vi "Serialize.vi"(7 "MsgSerializer":refnum<class "MsgSerializer.JSON.lvclass">, 8 "error in (no error)":errorcluster, 11 "Value":variant) -> (0 "error out":errorcluster, 3 "Serialized Message":string)   [LabVIEW 2020, in "Caraya.lvlib" / "MsgSerializer.JSON.lvclass"]
uses:
  MsgSerializer.JSON.lvclass
  <vilib>/Utility/VariantDataType/VariantType.lvlib
  Caraya.lvlib
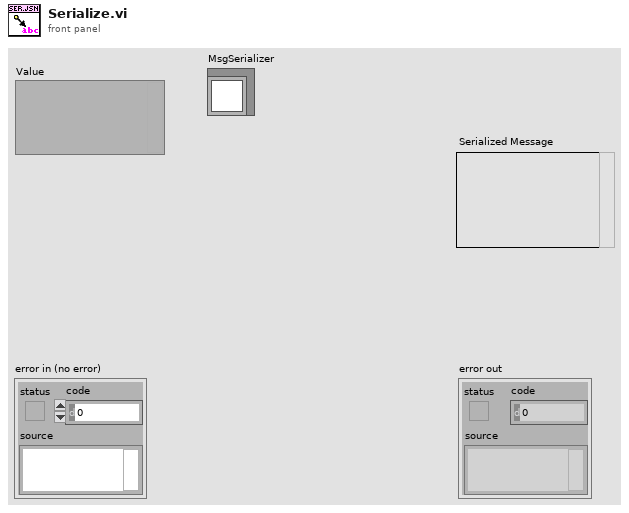
[diagram p1: front panel]
types:
  T1 = typedef "VariantType.lvlib/Type.ctl" = enum8{"Invalid Type", "Void", "I8", "I16", "I32", "I64", "U8", "U16", "U32", "U64", "Single Float", "Double Float", "Extended Float", "Single Complex", "Double Complex", "Extended Complex", "Enum U8", "Enum U16", "Enum U32", "Enum U64", "Single Float With Unit", "Double Float With Unit", "Extended Float With Unit", "Single Complex with Unit", "Double Complex with Unit", "Extended Complex with Unit", "Boolean", "String", "Path", "Picture", "Tag", "Array", "Cluster", "Variant", "LV Variant", "Waveform", "Timestamp", "Digital Waveform", "Digital Data", "ExpressData", "Refnum", "External Data", "VI", "Poly VI", "LabVIEW Class Instance", "Fixed Point"}
  T2 = typedef "TD_MDTFlavor.ctl" = enum16{"kUnknown", "OldDblWaveform", "I16Waveform", "DBLWaveform", "Unused(4)", "SGLWaveform", "Timestamp", "DigitalTable", "DigitalWaveform", "Dynamic Express", "ExtWaveform", "U8Waveform", "U16Waveform", "U32Waveform", "I8Waveform", "I32Waveform", "CSGWaveform", "CDBWaveform", "CXTWaveform", "I64Waveform", "U64Waveform"}
  T3 = typedef "VariantType.lvlib/RefnumType.ctl" = enum16{"NotARefnum", "UnknownRefnum", "Generic", "Datalog", "ByteStream", "Device", "Occurence", "TCPNetConnection", "Auto", "Menu", "Imaq", "Hardware", "DataSocket", "Visa", "IVI", "UDPNetConnection", "Notifier", "Queue", "Irda", "EventReg", "DotNet", "UserEvent", "Callback", "UNUSED_EMPTY_POSITION", "BlueToothNetConnection", "LVObjApp", "LVObjVI", "LVObjUnknown", "GenericClass", "UserDefinedRefnumTag", "DataValue", "RT FIFO", "TDMS File"}
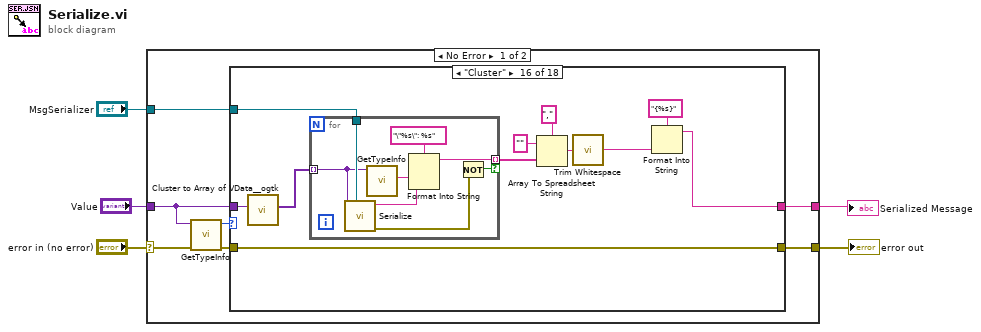
[diagram p0: block diagram]
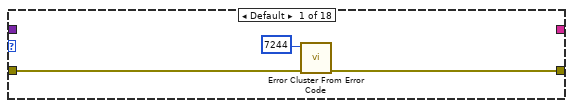
[diagram p2: hidden frame]
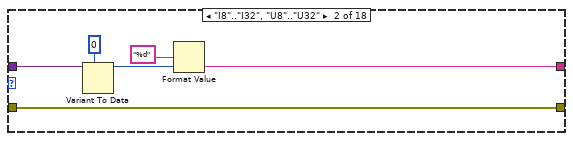
[diagram p3: hidden frame]
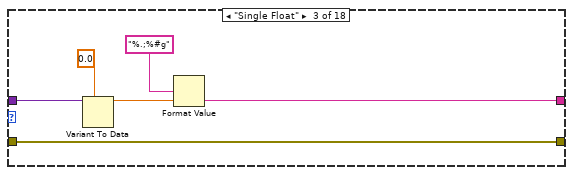
[diagram p4: hidden frame]
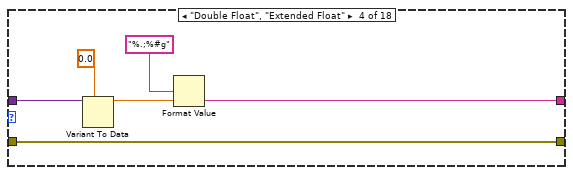
[diagram p5: hidden frame]
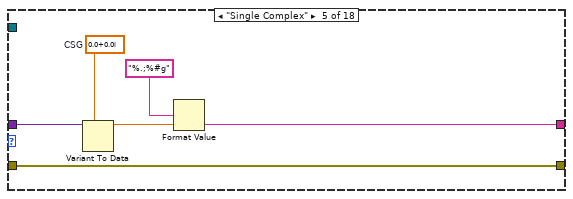
[diagram p6: hidden frame]
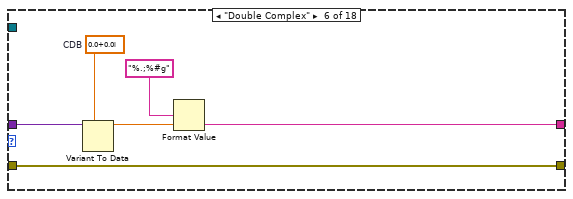
[diagram p7: hidden frame]
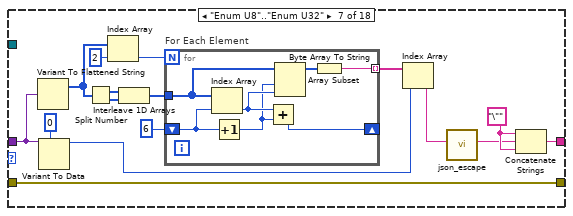
[diagram p8: hidden frame]
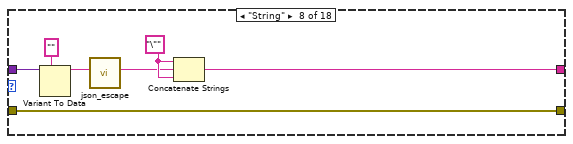
[diagram p9: hidden frame]
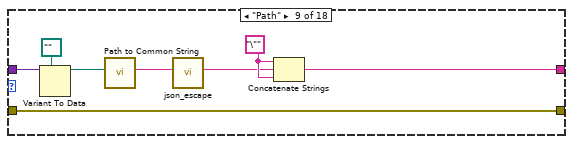
[diagram p10: hidden frame]
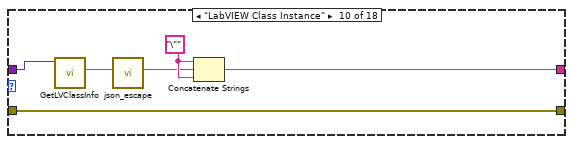
[diagram p11: hidden frame]
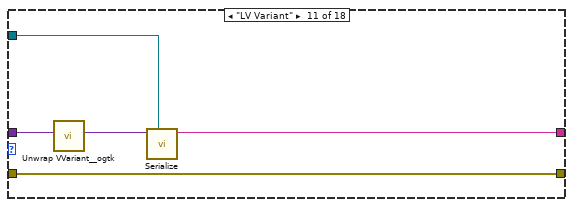
[diagram p12: hidden frame]
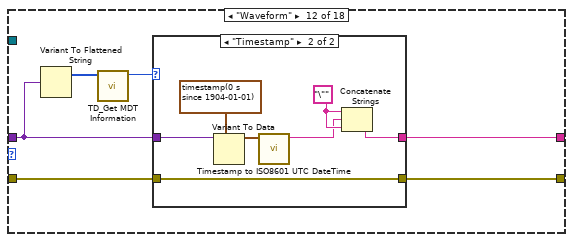
[diagram p13: hidden frame]
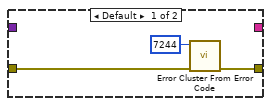
[diagram p14: hidden frame]
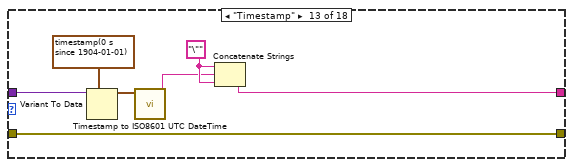
[diagram p15: hidden frame]
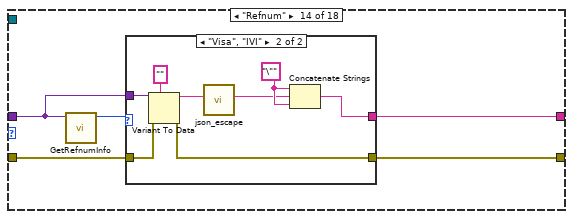
[diagram p16: hidden frame]
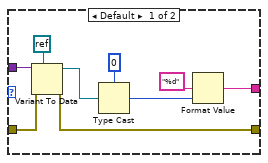
[diagram p17: hidden frame]
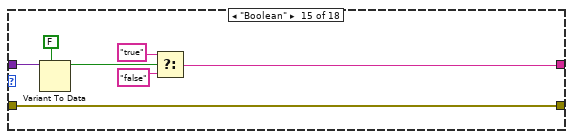
[diagram p18: hidden frame]
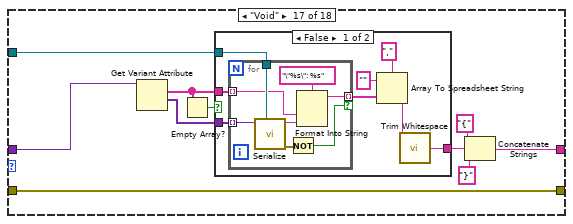
[diagram p19: hidden frame]
diagram:
  n1 = case shown="No Error" "error in (no error)" {
    selector: "error in (no error)" -> [w7 w208]
    tunnel: "MsgSerializer" -> [w12 _]
    tunnel: [w11 _] -> w4
    tunnel: "Value" -> [w10 _]
    tunnel: [w8 w208] -> w2
    frame No Error {
      n2 = call <vilib>:"GetTypeInfo.vi"("error in (no error)"=w7, "Variant"=w10) -> ("error out"=w6:errorcluster, "Type Enum"=w9:T1)  [unwired: 5 in, 3 out]
      n3 = case shown="\"Cluster\"" w9 {
        tunnel: [_ w17 w23 w29 w36 w42 w51 w73 w81 w89 w91 w95 w115 w120 w141 w153 w175 w198] -> w11
        tunnel: w10 -> [_ w21 w27 w33 w39 w45 w52 w74 w82 w87 w92 w98 w117 w121 w145 w150 w173 w194]
        tunnel: w12 -> [_ _ _ _ _ _ _ _ _ _ w90 _ _ _ _ w157 w174 w202]
        tunnel: w6 -> [w14 w16 w22 w28 w34 w40 w48 w71 w78 w86 w94 w97 w116 w119 w140 w149 w166 w192]
        tunnel: [w13 w16 w22 w28 w34 w40 w48 w71 w78 w86 w94 w96 w116 w118 w140 w149 w166 w192] -> w8
        frame Default {
          n4 = call <vilib>:"Error Cluster From Error Code.vi"("error in (no error)"=w14, "error code (0)"=7244) -> ("error out"=w13:errorcluster)  [unwired: 7 in]
        }
        frame "I8".."I32", "U8".."U32" {
          n5 = Variant To Data(type=i64 0, Variant=w21) -> (data=w20:i64)  [unwired: 1 in, 1 out]
          n6 = Format Value(format string="%d", value (0)=w20) -> (output string=w17:string)  [unwired: 1 in]
        }
        frame "Single Float" {
          n7 = Variant To Data(type=sgl 0.0, Variant=w27) -> (data=w26:sgl)  [unwired: 1 in, 1 out]
          n8 = Format Value(format string="%.;%#g", value (0)=w26) -> (output string=w23:string)  [unwired: 1 in]
        }
        frame "Double Float", "Extended Float" {
          n9 = Variant To Data(type=0.0, Variant=w33) -> (data=w32:dbl)  [unwired: 1 in, 1 out]
          n10 = Format Value(format string="%.;%#g", value (0)=w32) -> (output string=w29:string)  [unwired: 1 in]
        }
        frame "Single Complex" {
          w35 = csg 0.0+0.0i  # CSG
          n11 = Variant To Data(type=w35, Variant=w39) -> (data=w38:csg)  [unwired: 1 in, 1 out]
          n12 = Format Value(format string="%.;%#g", value (0)=w38) -> (output string=w36:string)  [unwired: 1 in]
        }
        frame "Double Complex" {
          w41 = cdb 0.0+0.0i  # CDB
          n13 = Variant To Data(type=w41, Variant=w45) -> (data=w44:cdb)  [unwired: 1 in, 1 out]
          n14 = Format Value(format string="%.;%#g", value (0)=w44) -> (output string=w42:string)  [unwired: 1 in]
        }
        frame "Enum U8".."Enum U32" {
          w50 = "\"" ("string")
          n15 = Variant To Flattened String(Variant=w52) -> (1:w53:i16[])  [unwired: 1 out]
          n16 = Variant To Data(type=u32 0, Variant=w52) -> (data=w49:u32)  [unwired: 1 in, 1 out]
          n17 = Split Number(x=w53) -> (hi(x)=w58:u8[], lo(x)=w57:u8[])
          n18 = Index Array(array=w53, index=2) -> (element=w60:i16)
          n19 = Interleave 1D Arrays(w58, w57) -> (w56:u8[])
          n20 = for "For Each Element" {
            N: w60 -> [_]
            shift-right: [w65] -> _
            shift-left: 6 ("index") -> [w68]
            tunnel: w56 -> [w66]
            tunnel: [w63] -> w54 mode=indexing
            n21 = Index Array(array=w66, index=w68) -> (element=w64:u8)
            n22 = Increment(x=w68) -> (x+1=w62:i32)
            n23 = Add(x=w64, y=w62) -> (x+y=w65:i32)
            n24 = Array Subset(array=w66, index=w62, length=w64) -> (w67:u8[])
            n25 = Byte Array To String(unsigned byte array=w67) -> (string=w63:string)
          }
          n26 = Index Array(array=w54, index=w49) -> (element=w47:string)
          n27 = call "json_escape.vi"("string"=w47) -> ("escaped string"=w46:string)  [unwired: 10 in]
          n28 = Concatenate Strings(w50, w46, w50) -> (w51:string)
        }
        frame "String" {
          w72 = "\"" ("string")
          n29 = Variant To Data(type="", Variant=w74) -> (data=w70:string)  [unwired: 1 in, 1 out]
          n30 = call "json_escape.vi"("string"=w70) -> ("escaped string"=w69:string)  [unwired: 10 in]
          n31 = Concatenate Strings(w72, w69, w72) -> (w73:string)
        }
        frame "Path" {
          w80 = "\"" ("string")
          n32 = Variant To Data(type=path "", Variant=w82) -> (data=w79:path)  [unwired: 1 in, 1 out]
          n33 = call "Path to Common String.vi"("specific path"=w79) -> ("common path"=w77:string)  [unwired: 10 in]
          n34 = call "json_escape.vi"("string"=w77) -> ("escaped string"=w76:string)  [unwired: 10 in]
          n35 = Concatenate Strings(w80, w76, w80) -> (w81:string)
        }
        frame "LabVIEW Class Instance" {
          w88 = "\"" ("string")
          n36 = call <vilib>:"GetLVClassInfo.vi"("Variant"=w87) -> ("LV Class File Name"=w85:string)  [unwired: 8 in, 2 out]
          n37 = call "json_escape.vi"("string"=w85) -> ("escaped string"=w84:string)  [unwired: 10 in]
          n38 = Concatenate Strings(w88, w84, w88) -> (w89:string)
        }
        frame "LV Variant" {
          n39 = call <userlib>:"Unwrap VVariant__ogtk.vi"("VVariant"=w92) -> ("Variant"=w93:variant)  [unwired: 9 in, 1 out]
          n40 = call-dynamic "Serialize.vi"("MsgSerializer"=w90, "Value"=w93) -> ("Serialized Message"=w91:string)  [unwired: 8 in, 1 out]
        }
        frame "Waveform" {
          n41 = Variant To Flattened String(Variant=w98) -> (1:w100:i16[])  [unwired: 1 out]
          n42 = call <vilib>:"TD_Get MDT Information.vi"("Type descriptor"=w100) -> ("MDT Flavor"=w99:T2)  [unwired: 9 in, 1 out]
          n43 = case shown="\"Timestamp\"" w99 {
            tunnel: w98 -> [_ w109]
            tunnel: [_ w106] -> w95
            tunnel: w97 -> [w102 w108]
            tunnel: [w103 w108] -> w96
            frame Default {
              n44 = call <vilib>:"Error Cluster From Error Code.vi"("error in (no error)"=w102, "error code (0)"=7244) -> ("error out"=w103:errorcluster)  [unwired: 7 in]
            }
            frame "Timestamp" {
              w107 = "\"" ("string")
              n45 = Variant To Data(type=timestamp(0 s since 1904-01-01) ("current time"), Variant=w109) -> (data=w105:timestamp)  [unwired: 1 in, 1 out]
              n46 = call <vilib>:"Timestamp to ISO8601 UTC DateTime.vi"("Timestamp (now)"=w105) -> ("ISO8601 UTC DateTime"=w104:string)  [unwired: 10 in]
              n47 = Concatenate Strings(w107, w104, w107) -> (w106:string)
            }
          }
        }
        frame "Timestamp" {
          w113 = "\"" ("string")
          n48 = Variant To Data(type=timestamp(0 s since 1904-01-01) ("current time"), Variant=w117) -> (data=w112:timestamp)  [unwired: 1 in, 1 out]
          n49 = call <vilib>:"Timestamp to ISO8601 UTC DateTime.vi"("Timestamp (now)"=w112) -> ("ISO8601 UTC DateTime"=w111:string)  [unwired: 10 in]
          n50 = Concatenate Strings(w113, w111, w113) -> (w115:string)
        }
        frame "Refnum" {
          n51 = call <vilib>:"GetRefnumInfo.vi"("Variant"=w121) -> ("ReferenceType"=w122:T3)  [unwired: 7 in, 3 out]
          n52 = case shown="\"Visa\", \"IVI\"" w122 {
            tunnel: w121 -> [w131 w137]
            tunnel: [w129 w136] -> w120
            tunnel: w119 -> [w128 w135]
            tunnel: [w127 w134] -> w118
            frame Default {
              n53 = Variant To Data(error in=w128, type=refnum<k0> refnum, Variant=w131) -> (data=w123:refnum<k0>, error out=w127:errorcluster)
              n54 = Type Cast(type=u32 0, x=w123) -> (*(type *) &x=w124:u32)
              n55 = Format Value(format string="%d", value (0)=w124) -> (output string=w129:string)  [unwired: 1 in]
            }
            frame "Visa", "IVI" {
              w138 = "\"" ("string")
              n56 = Variant To Data(error in=w135, type="", Variant=w137) -> (data=w133:string, error out=w134:errorcluster)
              n57 = call "json_escape.vi"("string"=w133) -> ("escaped string"=w132:string)  [unwired: 10 in]
              n58 = Concatenate Strings(w138, w132, w138) -> (w136:string)
            }
          }
        }
        frame "Boolean" {
          n59 = Variant To Data(type=FALSE, Variant=w145) -> (data=w142:bool)  [unwired: 1 in, 1 out]
          n60 = Select(t="true", s=w142, f="false") -> (s? t:f=w141:string)
        }
        frame "Cluster" {
          n61 = call <userlib>:"Cluster to Array of VData__ogtk.vi"("Cluster"=w150) -> ("Array of VData"=w147:variant[])  [unwired: 9 in, 1 out]
          n62 = for {
            tunnel: w147 -> [w161] mode=indexing
            tunnel: w157 -> [w164]
            tunnel: [w162] -> w148 mode=indexing if=w158
            n63 = call-dynamic "Serialize.vi"("MsgSerializer"=w164, "Value"=w161) -> ("error out"=w159:errorcluster, "Serialized Message"=w165:string)  [unwired: 8 in]
            n64 = call <vilib>:"GetTypeInfo.vi"("Variant"=w161) -> ("Name"=w160:string)  [unwired: 6 in, 4 out]
            n65 = Format Into String(format string="\"%s\": %s", w160, w165) -> (resulting string=w162:string)  [unwired: 2 in, 1 out]
            n66 = Not(x=w159) -> (.not. x?=w158:bool)
          }
          n67 = Array To Spreadsheet String(delimiter (Tab)=",", array=w148, 3:"" ("format string")) -> (spreadsheet string=w156:string)
          n68 = call <vilib>:"Trim Whitespace.vi"("string"=w156) -> ("trimmed string"=w155:string)  [unwired: 1 in]
          n69 = Format Into String(format string="{%s}", w155) -> (resulting string=w153:string)  [unwired: 2 in, 1 out]
        }
        frame "Void" {
          n70 = Get Variant Attribute(Variant=w173) -> (names=w171:string[], values=w170:variant[])  [unwired: 3 in, 2 out]
          n71 = Empty Array?(array=w171) -> (empty?=w172:bool)
          n72 = case shown="False" w172 {
            tunnel: w171 -> [w181 _]
            tunnel: w170 -> [w182 _]
            tunnel: w174 -> [w183 _]
            tunnel: [w176 _] -> w167
            frame False {
              n73 = for {
                tunnel: w183 -> [w191]
                tunnel: w182 -> [w190] mode=indexing
                tunnel: w181 -> [w189] mode=indexing
                tunnel: [w186] -> w177 mode=indexing if=w184
                n74 = call-dynamic "Serialize.vi"("MsgSerializer"=w191, "Value"=w190) -> ("error out"=w185:errorcluster, "Serialized Message"=w188:string)  [unwired: 8 in]
                n75 = Not(x=w185) -> (.not. x?=w184:bool)
                n76 = Format Into String(format string="\"%s\": %s", w189, w188) -> (resulting string=w186:string)  [unwired: 2 in, 1 out]
              }
              n77 = Array To Spreadsheet String(delimiter (Tab)=",", array=w177, 3:"" ("format string")) -> (spreadsheet string=w180:string)
              n78 = call <vilib>:"Trim Whitespace.vi"("string"=w180) -> ("trimmed string"=w176:string)  [unwired: 1 in]
            }
            frame True {
            }
          }
          n79 = Concatenate Strings("{" ("string"), w167, "}" ("format string")) -> (w175:string)
        }
        frame "Array" {
          n80 = call <userlib>:"Array to Array of VData__ogtk.vi"("MultiD Array"=w194) -> ("1D Array of Variants"=w193:variant[])  [unwired: 9 in, 1 out]
          n81 = for {
            tunnel: w193 -> [w206] mode=indexing
            tunnel: w202 -> [w207]
            tunnel: [w205] -> w195 mode=indexing if=w204
            n82 = call-dynamic "Serialize.vi"("MsgSerializer"=w207, "Value"=w206) -> ("error out"=w203:errorcluster, "Serialized Message"=w205:string)  [unwired: 8 in]
            n83 = Not(x=w203) -> (.not. x?=w204:bool)
          }
          n84 = Array To Spreadsheet String(delimiter (Tab)=",", array=w195, 3:"" ("format string")) -> (spreadsheet string=w201:string)
          n85 = call <vilib>:"Trim Whitespace.vi"("string"=w201) -> ("trimmed string"=w200:string)  [unwired: 1 in]
          n86 = Format Into String(format string="[%s]", w200) -> (resulting string=w198:string)  [unwired: 2 in, 1 out]
        }
      }
    }
    frame Error {
    }
  }
  "error out" <- w2
  "Serialized Message" <- w4
